vi "get result details.vi"(0 "test result":T1) -> (4 "test case":T2[](array[typedef]), 6 "Test Suites Atrributes":T14, 8 "test status":T3, 10 "test path":path, 15 "errors":T11[](array[typedef]))   [LabVIEW 2013]
uses:
  <vilib>/utf/common/utf_error_data.ctl
  <vilib>/utf/common/utf_error_type.ctl
  <vilib>/utf/common/utf_test_result.ctl
  <vilib>/utf/common/utf_test_result_testcase.ctl
  <vilib>/utf/common/utf_test_result_troll_new.ctl
  <vilib>/utf/common/utf_vector_result.ctl
  <vilib>/utf/common/utf_test_result_failure.ctl
  <vilib>/utf/common/utf_test_comparison_operators.ctl
  <vilib>/utf/common/utf_vi_tag.ctl
  <vilib>/utf/common/utf_test_result_input_data.ctl
  <vilib>/utf/common/utf_code_coverage.ctl
  <vilib>/NI/JUnit Results API/Controls/Test Suite Attribute Values.ctl
  <vilib>/utf/common/utf_test_result_testfile.ctl
  <vilib>/utf/common/utf_subvi_info.ctl
  <vilib>/NI/JUnit Results API/JUnit API.lvlib
  <vilib>/utf/NI_UnitTestFramework.lvlib
panel:
  out "error out":errorcluster
  in  "error in (no error)":errorcluster
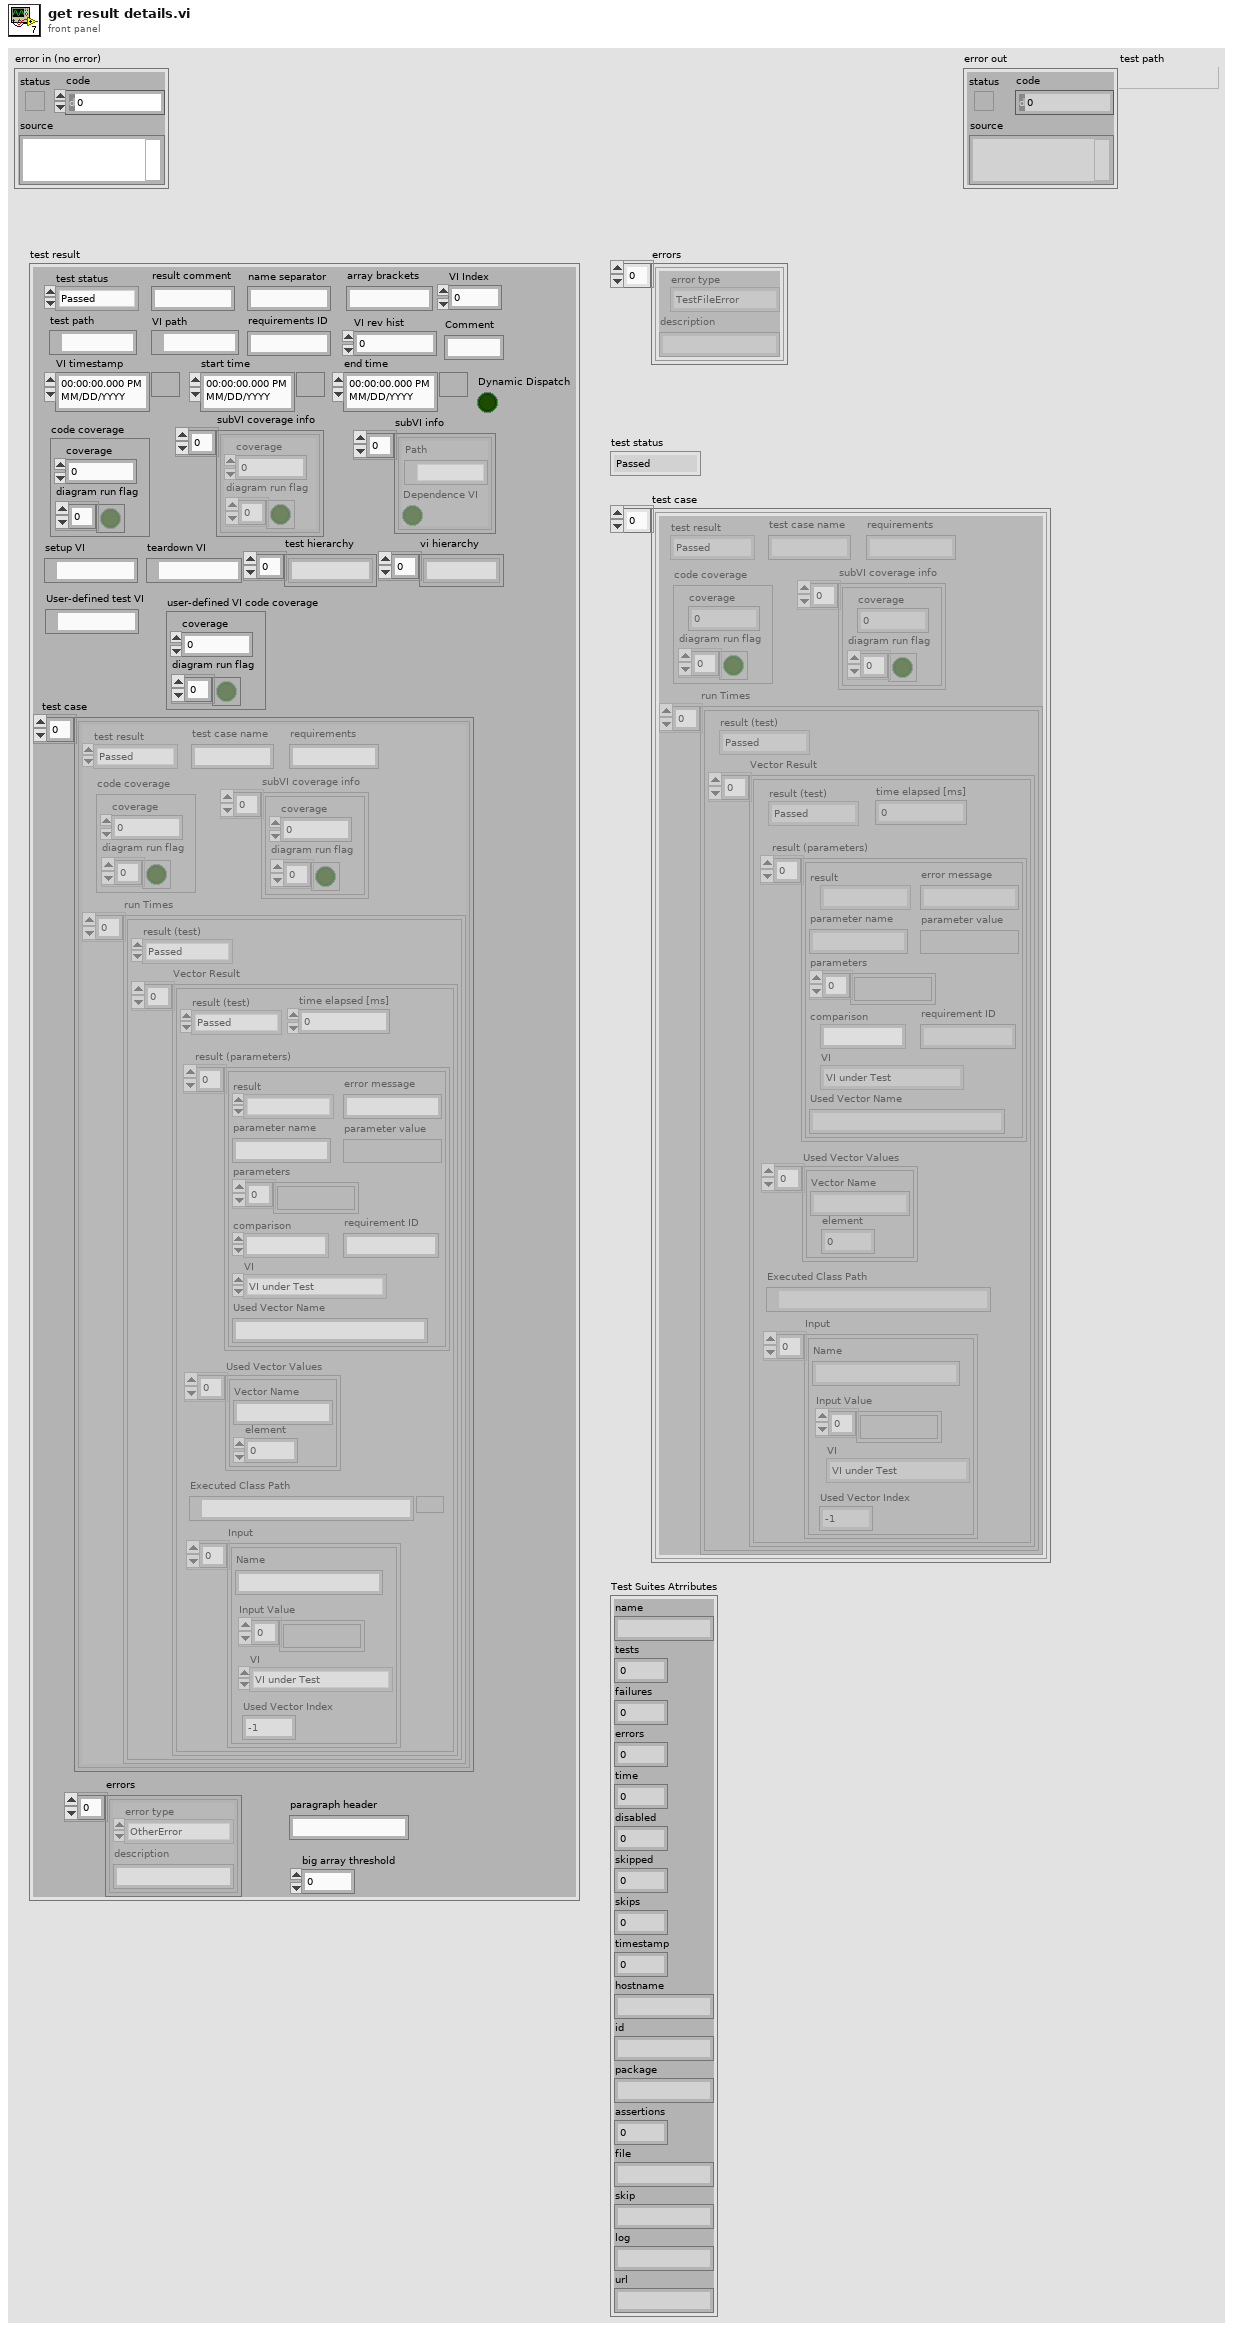
[diagram p1: front panel]
types:
  T1 = typedef "NI_UnitTestFramework.lvlib/utf_test_result_testfile.ctl" = cluster{"test case":T2[], "test status":T3, "test path":path, "setup VI":path, "teardown VI":path, "code coverage":T10, "start time":timestamp, "end time":timestamp, "test hierarchy":string[], "VI path":path, "VI timestamp":timestamp, "VI rev hist":i32, "requirements ID":string, "array brackets":string, "name separator":string, "errors":T11[], "paragraph header":string, "result comment":string, "vi hierarchy":string[], "subVI coverage info":T10[], "subVI info":T13[], "big array threshold":u32, "VI Index":i32, "Comment":string, "Dynamic Dispatch":bool, "User-defined test VI":path, "user-defined VI code coverage":T10}
  T2 = typedef "NI_UnitTestFramework.lvlib/utf_test_result_testcase.ctl" = cluster{"test result":T3, "run Times":T4[], "test case name":string, "requirements":string, "code coverage":T10, "subVI coverage info":T10[]}
  T3 = typedef "NI_UnitTestFramework.lvlib/utf_test_result.ctl" = enum16{"Passed", "Failed", "Error", "Skipped", "Not Processed"}
  T4 = typedef "NI_UnitTestFramework.lvlib/utf_test_result_troll_new.ctl" = cluster{"result (test)":T3, "Vector Result":T5[]}
  T5 = typedef "NI_UnitTestFramework.lvlib/utf_vector_result.ctl" = cluster{"time elapsed [ms]":u32, "result (test)":T3, "result (parameters)":T6[], "Used Vector Values":cluster{"Vector Name":string, "element":i32}[], "Executed Class Path":path, "Input":T9[]}
  T6 = typedef "NI_UnitTestFramework.lvlib/utf_test_result_failure.ctl" = cluster{"result":T3, "error message":string, "parameter name":string, "parameter value":variant, "parameters":variant[], "comparison":T7, "requirement ID":string, "VI":T8, "Used Vector Name":string}
  T7 = typedef "NI_UnitTestFramework.lvlib/utf_test_comparison_operators.ctl" = enum16{"=", "!=", ">", ">=", "<", "<=", "range", "symmetric tolerance", "asymmetric tolerance", "string contains", "string not contain", "array size", "string length", "array range", "by element", "array range (limit array)", "user-defined", "array contains", "array not contain", "vector length", "= (elm)", "!= (elm)", "= (case insensitive)", "!= (case insensitive)"}
  T8 = typedef "NI_UnitTestFramework.lvlib/utf_vi_tag.ctl" = enum16{"Setup VI", "VI under Test", "Teardown VI"}
  T9 = typedef "NI_UnitTestFramework.lvlib/utf_test_result_input_data.ctl" = cluster{"Name":string, "Input Value":variant[], "VI":T8, "Used Vector Index":i32}
  T10 = typedef "NI_UnitTestFramework.lvlib/utf_code_coverage.ctl" = cluster{"coverage":dbl, "diagram run flag":bool[]}
  T11 = typedef "NI_UnitTestFramework.lvlib/utf_error_data.ctl" = cluster{"error type":T12, "description":string}
  T12 = typedef "NI_UnitTestFramework.lvlib/utf_error_type.ctl" = enum16{"TestFileError", "VIError", "SetupVIError", "TearDownVIError", "OtherError"}
  T13 = typedef "NI_UnitTestFramework.lvlib/utf_subvi_info.ctl" = cluster{"Path":path, "Dependence VI":bool}
  T14 = typedef "JUnit API.lvlib/Test Suite Attribute Values.ctl" = cluster{"name":string, "tests":i32, "failures":i32, "errors":i32, "time":dbl, "disabled":i32, "skipped":i32, "skips":i32, "timestamp":dbl, "hostname":string, "id":string, "package":string, "assertions":i32, "file":string, "skip":string, "log":string, "url":string}
  T15 = typedef "NI_UnitTestFramework.lvlib/utf_test_properties.ctl" = cluster{"Test File Header":T16, "Test Values":T20[], "Setup Teardown Info":T24, "Setup Values":T20[], "Teardown Values":T20[], "Vector Info":cluster{"included vector files":path[], "vector array":T27[], "included and inherited vector files":path[]}}
  T16 = typedef "NI_UnitTestFramework.lvlib/utf_test_file_header.ctl" = cluster{"Test Name":string, "Comment":string, "VI Under Test":path, "Library":path, "Priority":u32, "Test Vector Execution":T17, "Array Brackets":string, "Requirements ID":string, "Skip for project window":bool, "Skip for palette VI":bool, "Repetitions":u32, "Set time-out":bool, "Time-out":u32, "Check Code Coverage":bool, "Minimum Code Coverage":u32, "User-defined Test":bool, "Name Separator":string, "User-defined Test VI":path, "Precision":u8, "Creation Type":T18, "Decimal separator":string, "Big Array Threshold":u32, "Save control names in normal format":bool, "Capture Input Value":bool, "Capture Output Value":bool, "Version":string, "Set automatic error handling":T19, "Remove breakpoints":bool}
  T17 = typedef "NI_UnitTestFramework.lvlib/utf_test_processing.ctl" = enum16{"None", "Linear", "Permutations"}
  T18 = typedef "NI_UnitTestFramework.lvlib/utf_test_creation_type.ctl" = enum16{"Include controls and indicators from connector pane", "Include controls and indicators from front panel", "Include controls and indicators from front panel as both input and output"}
  T19 = typedef "NI_UnitTestFramework.lvlib/utf_set_automatic_error_handling.ctl" = enum16{"As is", "Enable", "Disable"}
  T20 = typedef "NI_UnitTestFramework.lvlib/utf_test_values_cluster.ctl" = cluster{"Input Values Array":T21[], "Expected Values Array":T23[], "Test Case Name":string, "Test Case Comment":string}
  T21 = typedef "NI_UnitTestFramework.lvlib/utf_test_input_values.ctl" = cluster{"Name":string, "Data type":T22, "Input Value":variant[], "Default Flag":bool, "Requirements ID":string, "Array Type":i8, "Typedef Flag":bool, "Setup Flag":bool, "Terminal":string, "Global Variable":bool, "type information":variant, "Shared Variable":bool, "Use Vector":bool, "Vector Name":string, "Index":u8}
  T22 = typedef "VariantType.lvlib/Type.ctl" = enum8{"Invalid Type", "Void", "I8", "I16", "I32", "I64", "U8", "U16", "U32", "U64", "Single Float", "Double Float", "Extended Float", "Single Complex", "Double Complex", "Extended Complex", "Enum U8", "Enum U16", "Enum U32", "Enum U64", "Single Float With Unit", "Double Float With Unit", "Extended Float With Unit", "Single Complex with Unit", "Double Complex with Unit", "Extended Complex with Unit", "Boolean", "String", "Path", "Picture", "Tag", "Array", "Cluster", "Variant", "LV Variant", "Waveform", "Timestamp", "Digital Waveform", "Digital Data", "ExpressData", "Refnum", "External Data", "VI", "Poly VI", "LabVIEW Class Instance", "Fixed Point"}
  T23 = typedef "NI_UnitTestFramework.lvlib/utf_test_expected_values.ctl" = cluster{"Name":string, "Data type":T22, "Expected value":variant, "Check flag":bool, "Typedef Flag":bool, "Comparison":T7, "User-defined Comparison VI":path, "Requirements ID":string, "Array Type":i8, "by element":dbl, "Teardown Flag":bool, "Terminal":string, "Global Variable":bool, "type information":variant, "Shared Variable":bool, "By Element":bool, "Use Vector":bool, "Vector Name":string}
  T24 = typedef "NI_UnitTestFramework.lvlib/utf_setup_teardown_info.ctl" = cluster{"Setup VI":path, "Teardown VI":path, "Setup Data":T25[], "Teardown Data":T26[]}
  T25 = typedef "NI_UnitTestFramework.lvlib/utf_setup_info.ctl" = cluster{"Terminal":string, "Input":string}
  T26 = typedef "NI_UnitTestFramework.lvlib/utf_teardown_info.ctl" = cluster{"Terminal":string, "Output":string}
  T27 = typedef "NI_UnitTestFramework.lvlib/utf_vector_info.ctl" = cluster{"requirement ID":string, "file path":path, "Data type":T22, "append":string, "size":u64, "name":string, "vector edit type":enum16{"sequence", "linear"}, "values":variant[], "qualify name":string}
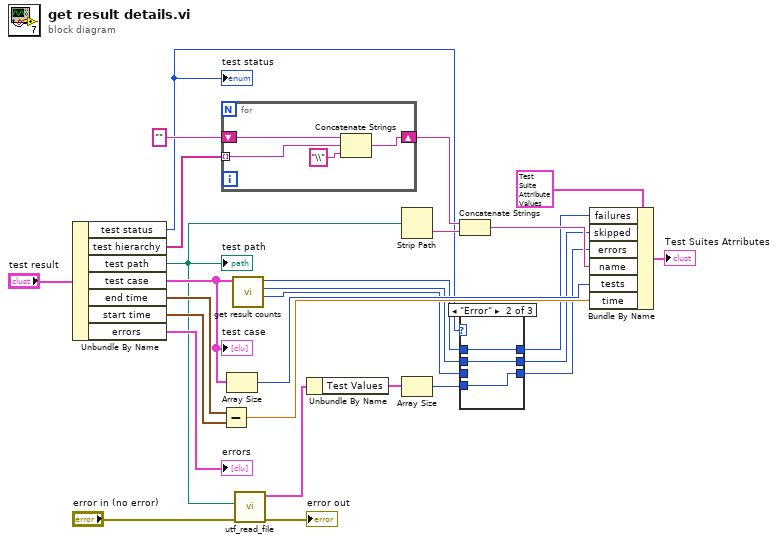
[diagram p0: block diagram]
diagram:
  n1 = Unbundle By Name("test result") -> ("test status"=w8:T3, "test hierarchy"=w17:string[], "test path"=w13:path, "test case"=w23:T2[], "end time"=w19:timestamp, "start time"=w20:timestamp, "errors"=→"errors":T11[])
  "test status" <- w8
  "test case" <- w23
  "test path" <- w13
  n2 = Subtract(x=w19, y=w20) -> (x-y=w22:dbl)
  n3 = for {
    tunnel: w17 -> [w30] mode=indexing
    shift-right: [w29] -> w25
    shift-left: "" -> [w31]
    n4 = Concatenate Strings(w31, w30, "\\" ("string")) -> (w29:string)
  }
  n5 = Array Size(array=w23) -> (size(s)=w21:i32)
  n6 = call "get result counts.vi"("test cases"=w23) -> ("error"=w5:i32, "skipped"=w6:i32, "failures"=w7:i32)  [unwired: 7 in, 1 out]
  n7 = call <vilib>:"utf_read_file.vi"("error in (no error)"="error in (no error)", "test file path"=w13) -> ("error out"=→"error out":errorcluster, "test specification out"=w12:T15)  [unwired: 5 in, 3 out]
  n8 = Unbundle By Name(w12) -> ("Test Values"=w9:T20[])
  n9 = Strip Path(path=w13) -> (name=w26:string)  [unwired: 1 out]
  n10 = Array Size(array=w9) -> (size(s)=w4:i32)
  n11 = Concatenate Strings(w25, w26) -> (w24:string)
  n12 = case shown="\"Error\"" w8 {
    tunnel: w7 -> [w34 w36 w39]
    tunnel: w6 -> [w33 w35 _]
    tunnel: w5 -> [w32 _ w38]
    tunnel: w4 -> [_ w37 w40]
    tunnel: [w34 w36 w39] -> w3
    tunnel: [w33 w35 w40] -> w2
    tunnel: [w32 w37 w38] -> w1
    frame "Passed", Default {
    }
    frame "Error" {
    }
    frame "Skipped" {
    }
  }
  n13 = Bundle By Name(cluster=T14 {"name"="", "tests"=0, "failures"=0, "errors"=0, "time"=0.0, "disabled"=0, "skipped"=0, "skips"=0, "timestamp"=0.0, "hostname"="", "id"="", "package"="", "assertions"=0, "file"="", "skip"="", "log"="", "url"=""} ("Test Suites Atrributes"), "failures"=w3, "skipped"=w2, "errors"=w1, "name"=w24, "tests"=w21, "time"=w22) -> (→"Test Suites Atrributes":T14)
